vi "process.vi"(8 "error in":errorcluster, 9 "result allocation":T1, 10 "data to process":T1, 11 "module in":refnum<class "tag bus processing plugin module.lvclass">) -> (0 "error out":errorcluster, 1 "result data":T1, 2 "processing allocation":T1, 3 "module out":refnum<class "tag bus processing plugin module.lvclass">)   [LabVIEW 2013, in "tag bus processing plugin module.lvclass"]
doc: "Provides an interface for information processing by a module at runtime. While this interface performs no operations, a child should provide an override which may process data in any manner necessary."
uses:
  tag bus processing plugin module.lvclass
  <vilib>/NI/Tag Bus/table/data table.ctl
  <vilib>/NI/Tag Bus/table/data polymorphs/read one/read Double.vi
  <vilib>/NI/Tag Bus/table/data polymorphs/write one/write Double.vi
  <vilib>/NI/Tag Bus/table/data table.lvlib
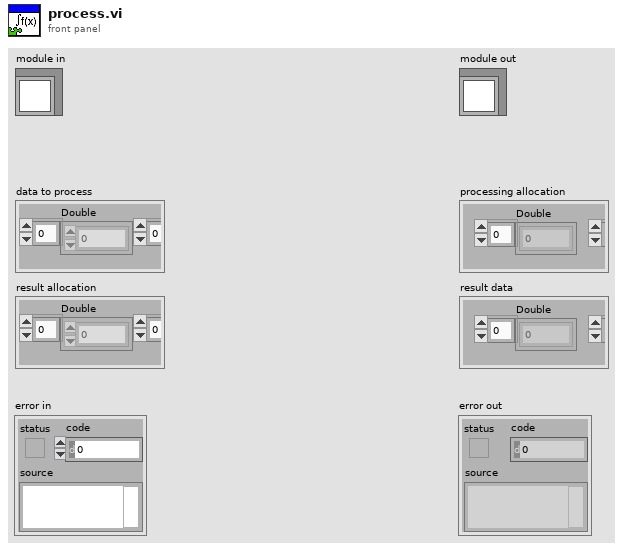
[diagram p1: front panel]
types:
  T1 = typedef "tag bus.lvlib/data table.lvlib/data table.ctl" = cluster{"Double":dbl[], "Single":sgl[], "I64":i64[], "I32":i32[], "I16":i16[], "I8":i8[], "U64":u64[], "U32":u32[], "U16":u16[], "U8":u8[], "Boolean":bool[], "String":string[], "Array of Double":cluster{"DBL Array":dbl[]}[], "Array of Single":cluster{"SGL Array":sgl[]}[], "Array of I64":cluster{"I64 Array":i64[]}[], "Array of I32":cluster{"I32 Array":i32[]}[], "Array of I16":cluster{"I16 Array":i16[]}[], "Array of I8":cluster{"I8 Array":i8[]}[], "Array of U64":cluster{"U64 Array":u64[]}[], "Array of U32":cluster{"U32 Array":u32[]}[], "Array of U16":cluster{"U16 Array":u16[]}[], "Array of U8":cluster{"U8 Array":u8[]}[], "Array of Boolean":cluster{"Boolean Array":bool[]}[], "Array of String":cluster{"String Array":string[]}[]}
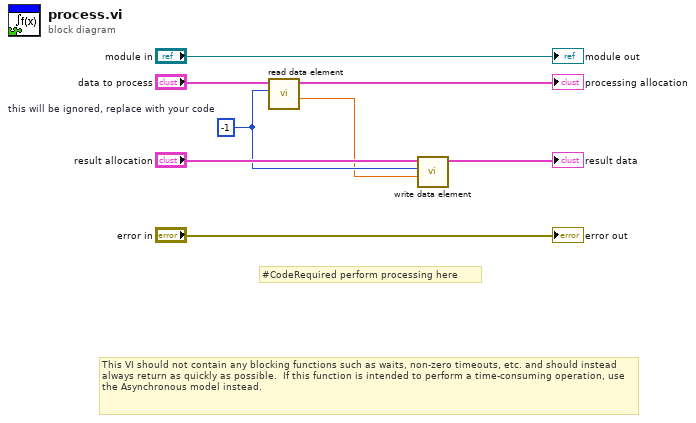
[diagram p0: block diagram]
diagram:
  w2 = -1  # this will be ignored, replace with your code
  # "#CodeRequired perform processing here"
  # "This VI should not contain any blocking functions such as waits, non-zero timeouts, etc. and should instead always return as quickly as possible.  If this function is intended to perform a time-consuming operation, use the Asynchronous model instead."
  n1 = call-poly <vilib>:"read data element.vi"("index"=w2, "data table in"="data to process") -> ("value"=w1:dbl, "data table out"=→"processing allocation":T1)  [unwired: 8 in]
  n2 = call-poly <vilib>:"write data element.vi"("value"=w1, "index"=w2, "data table in"="result allocation") -> ("data table out"=→"result data":T1)  [unwired: 8 in]
  "error out" <- "error in"
  "module out" <- "module in"
